vi "LVCAM Destroy Self.vi"(11 "Self Actor in":refnum<class "Self Actor.lvclass">) -> (0 "error out":errorcluster, 1 "Destroyed Self?":bool, 3 "Self Actor out":refnum<class "Self Actor.lvclass">)   [LabVIEW 2021, in "LVCAM.lvlib" / "Self Actor.lvclass"]
uses:
  Self Actor.lvclass
  C:/PPLs/LabVIEW-Composed-Actor-Model-LVCAM/LabVIEW-Composed-Actor-Model-LVCAM/LVCAM/LVCAM/LVCAM/LVCAM.lvclass
  State.ctl
  Self Actor.lvclass/Self Actor.ctl
  Msgs/LVCAM Destroy Self/LVCAM Destroy Self Msg/LVCAM Destroy Self Msg.lvclass
  C:/PPLs/LabVIEW-Composed-Actor-Model-LVCAM/LabVIEW-Composed-Actor-Model-LVCAM/LVCAM/LVCAM/Msg/Msg.lvclass
  Msgs/LVCAM Nest Destroyed/LVCAM Nest Destroyed Msg/LVCAM Nest Destroyed Msg.lvclass
  Nest Msg Send.vi
  Call Msg Send.vi
  C:/PPLs/LabVIEW-Composed-Actor-Model-LVCAM/LabVIEW-Composed-Actor-Model-LVCAM/LVCAM/Msgs/LVCAM Create Nest/LVCAM Create Nest/LVCAM Create Nest.lvclass
  C:/PPLs/LabVIEW-Composed-Actor-Model-LVCAM/LabVIEW-Composed-Actor-Model-LVCAM/LVCAM/Msgs/LVCAM Destroy Self/LVCAM Destroy Self/LVCAM Destroy Self.lvclass
  C:/PPLs/LabVIEW-Composed-Actor-Model-LVCAM/LabVIEW-Composed-Actor-Model-LVCAM/LVCAM/Msgs/LVCAM Nest Destroyed/LVCAM Nest Destroyed/LVCAM Nest Destroyed.lvclass
  C:/PPLs/LabVIEW-Composed-Actor-Model-LVCAM/LabVIEW-Composed-Actor-Model-LVCAM/LVCAM/LVCAM/LVCAM Msg Drop/LVCAM Msg Drop.lvclass
  C:/PPLs/LabVIEW-Composed-Actor-Model-LVCAM/LabVIEW-Composed-Actor-Model-LVCAM/LVCAM/LVCAM/LVCAM Msg Receive/LVCAM Msg Receive.lvclass
  C:/PPLs/LabVIEW-Composed-Actor-Model-LVCAM/LabVIEW-Composed-Actor-Model-LVCAM/LVCAM/LVCAM/LVCAM Propagate Error/LVCAM Propagate Error.lvclass
  C:/PPLs/LabVIEW-Composed-Actor-Model-LVCAM/LabVIEW-Composed-Actor-Model-LVCAM/LVCAM/LVCAM/LVCAM Write Self Actor/LVCAM Write Self Actor.lvclass
  C:/PPLs/LabVIEW-Composed-Actor-Model-LVCAM/LabVIEW-Composed-Actor-Model-LVCAM/LVCAM/LVCAM/Self Actor/Self Actor.lvclass
  C:/PPLs/LabVIEW-Composed-Actor-Model-LVCAM/LabVIEW-Composed-Actor-Model-LVCAM/LVCAM/Msgs/LVCAM Destroy Self/LVCAM Destroy Self Msg/LVCAM Destroy Self Msg.lvclass
  C:/PPLs/LabVIEW-Composed-Actor-Model-LVCAM/LabVIEW-Composed-Actor-Model-LVCAM/LVCAM/Msgs/LVCAM Nest Destroyed/LVCAM Nest Destroyed Msg/LVCAM Nest Destroyed Msg.lvclass
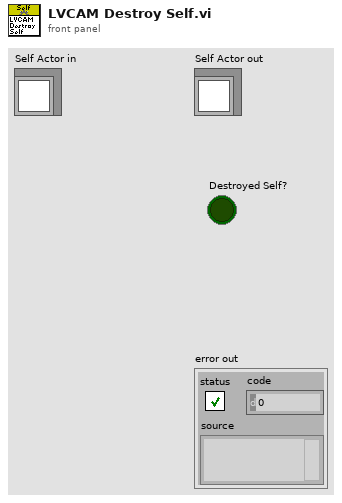
[diagram p1: front panel]
types:
  T1 = typedef "LVCAM.lvlib/Self Actor.lvclass/State.ctl" = enum16{"Safe Msging", "Destroying Self"}
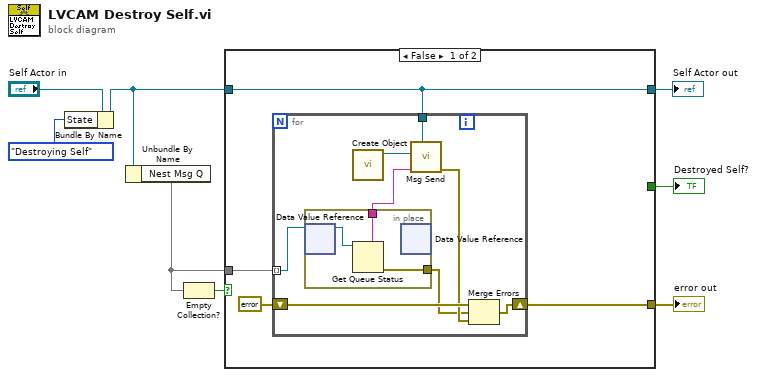
[diagram p0: block diagram]
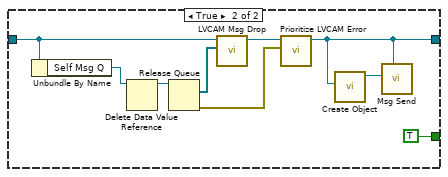
[diagram p2: hidden frame]
diagram:
  n1 = Bundle By Name(cluster="Self Actor in", "State"=State."Destroying Self") -> (w2:refnum<class "Self Actor.lvclass">)
  n2 = Unbundle By Name(w2) -> ("Nest Msg Q"=w5:set{refnum<data-value>})
  n3 = Empty Collection?(1:w5) -> (0:w6:bool)
  n4 = case shown="False" w6 {
    tunnel: w5 -> [w12 _]
    tunnel: [w11 _] -> w3
    tunnel: [_ TRUE ("Destroyed Self?")] -> w4
    tunnel: w2 -> [w9 w32]
    tunnel: [w9 w29] -> w1
    frame False {
      n5 = for {
        tunnel: w12 -> [w14] mode=indexing
        shift-right: [w20] -> w11
        shift-left: errorcluster {"status"=FALSE, "code"=0, "source"=""} ("error out") -> [w19]
        tunnel: w9 -> [w16]
        n6 = in-place {
          in-place-border: [w22] -> w15
          in-place-border: [w21] -> w13
          n7 = in-place-dvr #1(w14) -> (w23:refnum<queue>)  [unwired: 1 out]
          n8 = Get Queue Status(queue=w23) -> (queue name=w21:string, error out=w22:errorcluster)  [unwired: 2 in, 6 out]
          n9 = in-place-dvr #1() -> ()  [unwired: 1 in, 2 out]
        }
        n10 = call "Create Object.vi"() -> ("LVCAM Destroy Self Msg out"=w17:refnum<class "LVCAM Destroy Self Msg.lvclass">)  [unwired: 11 in]
        n11 = call-poly "Msg Send.vi"("Self Actor"=w16, "Alias"=w13, "Msg"=w17) -> ("error out"=w18:errorcluster)  [unwired: 7 in, 1 out]
        n12 = Merge Errors(w19, w15, w18) -> (w20:errorcluster)
      }
    }
    frame True {
      n13 = Unbundle By Name(w32) -> ("Self Msg Q"=w25:refnum<data-value>)
      n14 = Delete Data Value Reference(data value reference=w25) -> (data value=w24:refnum<queue>)  [unwired: 1 in, 1 out]
      n15 = Release Queue(queue=w24) -> (remaining elements=w26:refnum<class "Msg.lvclass">[], error out=w27:errorcluster)  [unwired: 2 in, 1 out]
      n16 = call-dynamic "LVCAM Msg Drop.vi"("Remaining Elements"=w26, "Self Actor in"=w32) -> ("Self Actor out"=w30:refnum<class "Self Actor.lvclass">)  [unwired: 9 in]
      n17 = call "Prioritize LVCAM Error.vi"("Error from LVCAM"=w27, "Self Actor in"=w30) -> ("Self Actor out"=w29:refnum<class "Self Actor.lvclass">)  [unwired: 9 in]
      n18 = call "Create Object.vi"("Nest Actor"=w29) -> ("LVCAM Nest Destroyed Msg out"=w28:refnum<class "LVCAM Nest Destroyed Msg.lvclass">)  [unwired: 10 in]
      n19 = call-poly "Msg Send.vi"("Self Actor"=w29, "Msg"=w28) -> ()  [unwired: 9 in, 1 out]
    }
  }
  "error out" <- w3
  "Self Actor out" <- w1
  "Destroyed Self?" <- w4
